vi "example_2010.vi"() -> ()   [LabVIEW 2010]
uses:
  <vilib>/Analysis/NI_AALPro.lvlib
  <vilib>/Analysis/NI_AALBase.lvlib
  <vilib>/Analysis/baseanly.llb/Mean (DBL).vi
panel:
  out "MAE Least Square":dbl format="%0.2f"
  out "MAE Theil-Sen":dbl format="%0.2f"
  out "intercept":dbl
  out "slope":dbl
  out "XY Graph":cluster{dbl[], dbl[]}[](graph)
  out "b":dbl format="%.6g"
  out "m":dbl format="%.6g"
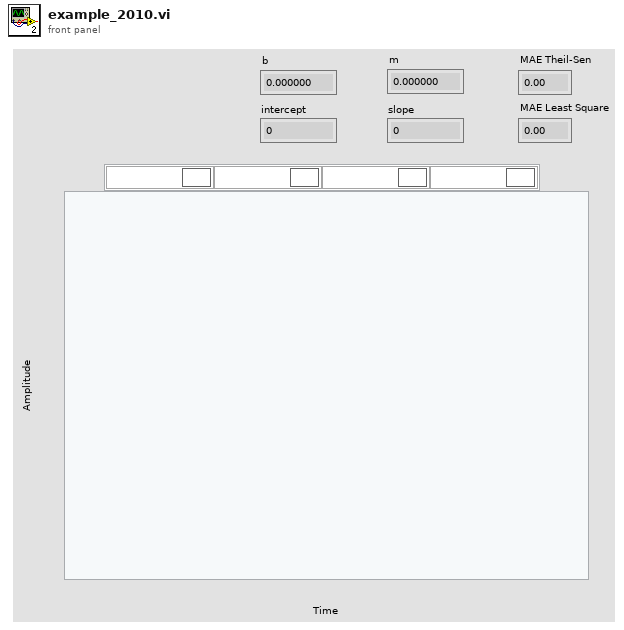
[diagram p1: front panel]
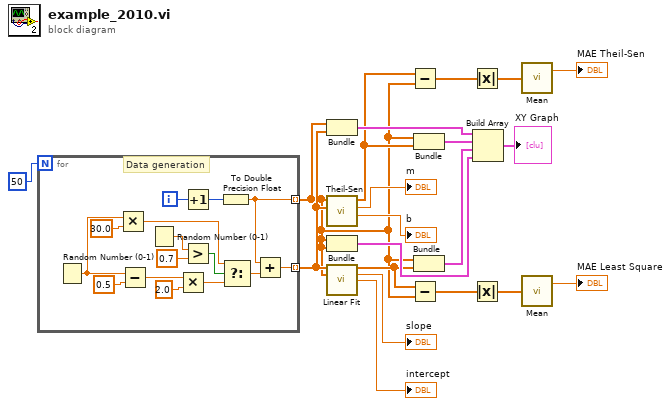
[diagram p0: block diagram]
diagram:
  n1 = for {
    N: 50 -> [_]
    tunnel: [w30] -> w1 mode=indexing
    tunnel: [w33] -> w8 mode=indexing
    i -> [w32]
    # "Data generation"
    n2 = Random Number (0-1)() -> (number: 0 to 1=w23:dbl)
    n3 = Multiply(x=w23, y=30.0 ("t")) -> (x*y=w22:dbl)
    n4 = Subtract(x=w23, y=0.5) -> (x-y=w35:dbl)
    n5 = Random Number (0-1)() -> (number: 0 to 1=w29:dbl)
    n6 = Multiply(x=w35, y=2.0) -> (x*y=w26:dbl)
    n7 = Increment(x=w32) -> (x+1=w31:i32)
    n8 = Greater?(x=w29, y=0.7) -> (0:w25:bool)
    n9 = To Double Precision Float(number=w31) -> (double precision float=w30:dbl)
    n10 = Select(t=w22, s=w25, f=w26) -> (s? t:f=w21:dbl)
    n11 = Add(x=w30, y=w21) -> (x+y=w33:dbl)
  }
  n12 = Bundle(w1, w8) -> (w19:cluster{dbl[], dbl[]})  [unwired: 1 in]
  n13 = call "Theil-Sen.vi"("input_Y"=w8, "input_X"=w1) -> ("b"=→"b":dbl, "m"=→"m":dbl, "output_Y"=w10:dbl[])  [unwired: 4 in, 1 out]
  n14 = Bundle(w1, w1) -> (w16:cluster{dbl[], dbl[]})  [unwired: 1 in]
  n15 = call <vilib>:"Linear Fit.vi"("Y"=w8, "X"=w1) -> ("Best Linear Fit"=w9:dbl[], "slope"=→"slope":dbl, "intercept"=→"intercept":dbl)  [unwired: 9 in, 2 out]
  n16 = Subtract(x=w10, y=w1) -> (x-y=w7:dbl[])
  n17 = Subtract(x=w9, y=w1) -> (x-y=w6:dbl[])
  n18 = Bundle(w1, "output_Y"=w10) -> (w18:cluster{dbl[], "output_Y":dbl[]})  [unwired: 1 in]
  n19 = Bundle(w1, "Best Linear Fit"=w9) -> (w15:cluster{dbl[], "Best Linear Fit":dbl[]})  [unwired: 1 in]
  n20 = Absolute Value(x=w7) -> (abs(x)=w5:dbl[])
  n21 = Absolute Value(x=w6) -> (abs(x)=w4:dbl[])
  n22 = Build Array(w19, w18, w15, w16) -> (→"XY Graph":cluster{dbl[], "Best Linear Fit":dbl[]}[])
  n23 = call-poly <vilib>:"Mean.vi"("X"=w5) -> ("mean"=→"MAE Theil-Sen":dbl)  [unwired: 1 out]
  n24 = call-poly <vilib>:"Mean.vi"("X"=w4) -> ("mean"=→"MAE Least Square":dbl)  [unwired: 1 out]
